vi "Load TLV File.vi"(8 "error in (no error)":errorcluster, 10 "TLV Path":path, 11 "object in":refnum<class "CAN IO.lvclass">) -> (0 "error out":errorcluster, 3 "object out":refnum<class "CAN IO.lvclass">)   [LabVIEW 2013, in "CAN IO.lvclass"]
uses:
  CAN IO.lvclass
panel:
  in  "TLV file ref":refnum<file>
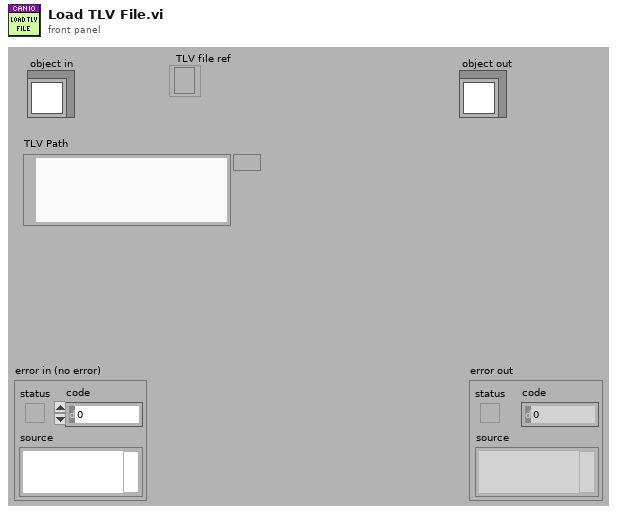
[diagram p1: front panel]
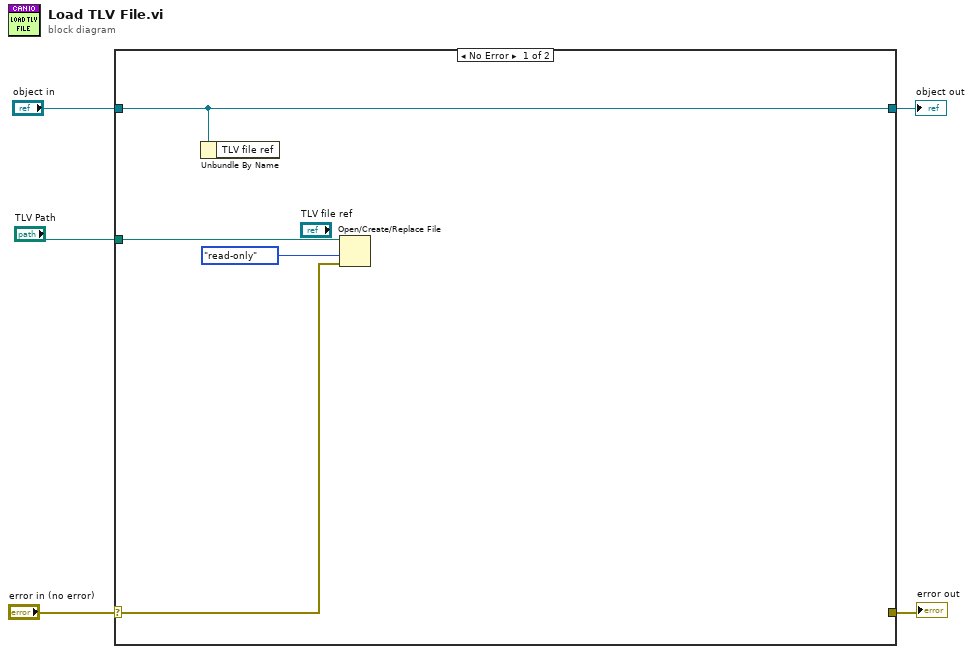
[diagram p0: block diagram]
diagram:
  n1 = case shown="No Error" "error in (no error)" {
    selector: "error in (no error)" -> [w6 w11]
    tunnel: [_ w11] -> w4
    tunnel: [w9 w10] -> w2
    tunnel: "object in" -> [w9 w10]
    tunnel: "TLV Path" -> [w8 _]
    frame No Error {
      n2 = Unbundle By Name(w9) -> ()  [unwired: 1 out]
      n3 = Open/Create/Replace File(file path (use dialog)=w8, error in=w6, access (0:read/write)=enum16{"read/write", "read-only", "write-only"}."read-only") -> ()  [unwired: 3 in, 3 out]
    }
    frame Error {
    }
  }
  "error out" <- w4
  "object out" <- w2
